vi "Waveform Attribute, Copy All Atttributes.vi"(6 "error in":errorcluster, 8 "src waveform":waveform(dbl)={"t0"=timestamp(3473168073.631 s since 1904-01-01), "dt"=1e-08, "Y"=[], "attributes"=variant("Average Size"=variant(dbl 15.0), "Frequency (Hz)"=variant(dbl 1997.9906429610444), "NSamp"=variant(dbl 400000.0), "Recvy Amp (mA)"=variant(dbl 5.267865023873527), "Recvy Amp (mV)"=variant(dbl 2633.932511936763), "Recvy Frequency (Hz)"=variant(dbl 1998.1395072914302), "Recvy Pulse Width (us)"=variant(dbl 12.427603778839112), "Recvy Trigger (s)"=variant(dbl 0.00043972), "Resistance (ohms)"=variant(dbl 500.0), "Samp Freq (MHz)"=variant(dbl 100.0), "Stim Amp (mA)"=variant(dbl -4.607747165232184), "Stim Amp (mV)"=variant(dbl -2303.873582616092), "Stim Frequency (Hz)"=variant(dbl 1997.8417786306586), "Stim Pulse Width (us)"=variant(dbl 12.076313257217407), "Stim Trigger (s)"=variant(dbl 0.00041185), "dt (us)"=variant(dbl 0.01))}, 9 "dst waveform":waveform(dbl)={"t0"=timestamp(3473168073.631 s since 1904-01-01), "dt"=1e-08, "Y"=[1.0, 2.0, 3.0], "attributes"=variant("Average Size"=variant(dbl 15.0), "Frequency (Hz)"=variant(dbl 1997.9906429610444), "NSamp"=variant(dbl 400000.0), "Recvy Amp (mA)"=variant(dbl 5.267865023873527), "Recvy Amp (mV)"=variant(dbl 2633.932511936763), "Recvy Frequency (Hz)"=variant(dbl 1998.1395072914302), "Recvy Pulse Width (us)"=variant(dbl 12.427603778839112), "Recvy Trigger (s)"=variant(dbl 0.00043972), "Resistance (ohms)"=variant(dbl 500.0), "Samp Freq (MHz)"=variant(dbl 100.0), "Stim Amp (mA)"=variant(dbl -4.607747165232184), "Stim Amp (mV)"=variant(dbl -2303.873582616092), "Stim Frequency (Hz)"=variant(dbl 1997.8417786306586), "Stim Pulse Width (us)"=variant(dbl 12.076313257217407), "Stim Trigger (s)"=variant(dbl 0.00041185), "dt (us)"=variant(dbl 0.01))}) -> (0 "error out":errorcluster, 1 "Attribute Count":i32=-1, 2 "src waveform dup":waveform(dbl)={"t0"=timestamp(25200.631000162026 s since 1904-01-01), "dt"=nan, "Y"=[]}, 3 "dst waveform out":waveform(dbl)={"t0"=timestamp(25200.631000162026 s since 1904-01-01), "dt"=nan, "Y"=[]})   [LabVIEW 2010]
doc: "This function copies all waveform attributes (as variant data) from the source waveform to the destination waveform.\n\nThe LabVIEW Get Waveform Attribute and Set Waveform Attribute VIs are used to transfer the data."
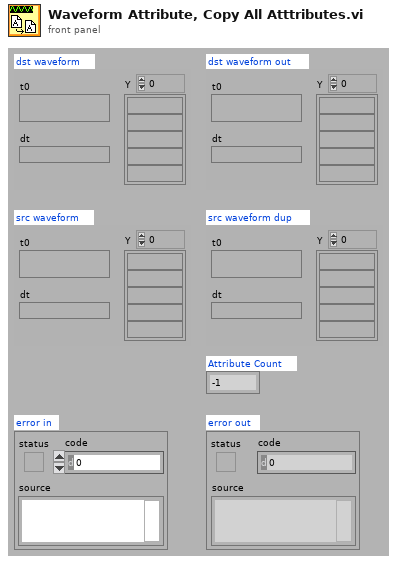
[diagram p1: front panel]
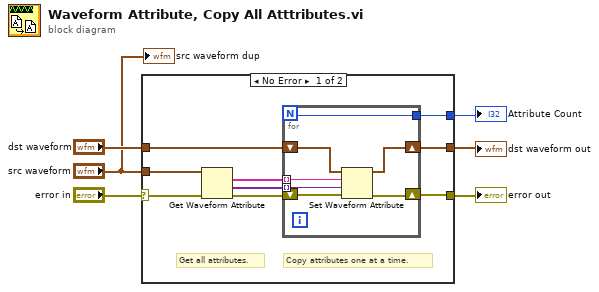
[diagram p0: block diagram]
diagram:
  n1 = case shown="No Error" "error in" {
    selector: "error in" -> [w14 w23]
    tunnel: "src waveform" -> [w15 _]
    tunnel: [w13 w23] -> w5
    tunnel: "dst waveform" -> [w8 _]
    tunnel: [w9 _] -> w3
    tunnel: [w7 _] -> w2
    frame No Error {
      # "Copy attributes one at a time."
      # "Get all attributes."
      n2 = Get Waveform Attribute(4:w14, 7:w15) -> (0:w12:errorcluster, 1:w10:variant[], 2:w11:string[])  [unwired: 2 in, 1 out]
      n3 = for {
        N -> [w16]
        shift-right: [w22] -> w13
        shift-left: w12 -> [w21]
        tunnel: w11 -> [w20] mode=indexing
        tunnel: w10 -> [w19] mode=indexing
        shift-right: [w18] -> w9
        shift-left: w8 -> [w17]
        tunnel: [w16] -> w7
        n4 = Set Waveform Attribute(4:w21, 5:w19, 6:w20, 7:w17) -> (0:w22:errorcluster, 3:w18:waveform(dbl))  [unwired: 1 out]
      }
    }
    frame Error {
    }
  }
  "error out" <- w5
  "dst waveform out" <- w3
  "Attribute Count" <- w2
  "src waveform dup" <- "src waveform"
